vi "Main.vi"(11 "Module Admin":refnum<class "Delacor_lib_QMH_Module Admin.lvclass">) -> ()   [LabVIEW 2021, in "PS.lvlib"]
doc: "This template is based off of the Queued Message Handler design pattern and the Queued Message Handler project template that ships with LabVIEW.\n\nThe main difference is that the queue is private to this module and communication between modules is performed via Broadcast and Request events.\n\nRequest events are wrapped in public API methods and are handled in the Event Handling Loop (EHL) of this VI. Any module can register for Broadcast events sent by this module. The EHL generates messages based on user interface actions.\n\nThe Message Handling Loop (MHL) processes messages generated by the EHL, or by other messages. The messages are string values, so new messages can be added easily to the Message Cases case structure in the MHL. Each message cluster can also provide an optional value for Message Data, which is a variant that can be converted to whatever message-specific data is required.\n_____\nBased on Delacor QMH Project Template 5.0.0.82.\n\n<b>Note:</b> This VI was modified by the <b>Validate DQMH Module</b> tool to add a 'Panel Hidden' status updated broadcast to the Panel Close? event when External Launch = TRUE.\n\n<b>Note:</b> This VI was modified by the <b>Validate DQMH Module</b> tool to add a call to the Error Reported VI at the end of the 'Exit' MHL frame."
uses:
  PS.lvlib
  <vilib>/Delacor/Delacor QMH/Libraries/Module Admin_class/Delacor_lib_QMH_Module Admin.lvclass
  td_en_pstype.ctl
  Classes/PS/PS.lvclass
  <vilib>/Delacor/Delacor QMH/Libraries/Message Queue_class/Delacor_lib_QMH_Message Queue.lvclass/Delacor_lib_QMH_Message Queue.ctl
  Stop Argument--cluster.ctl
  <vilib>/Delacor/Delacor QMH/Libraries/Module Admin_class/Delacor_lib_QMH_Module Admin.lvclass/Delacor_lib_QMH_Module Admin.ctl
  Set Power Supply Argument--cluster.ctl
  Set Voltage Argument--cluster.ctl
  Set Current Argument--cluster.ctl
  Set Output Argument--cluster.ctl
  Open Argument--cluster.ctl
  Open (Reply Payload)--cluster.ctl
  Close Argument--cluster.ctl
  Close (Reply Payload)--cluster.ctl
  Get PS Data Argument--cluster.ctl
  Get PS Data (Reply Payload)--cluster.ctl
  Load in SubPane Argument--cluster.ctl
  UnLoad SubPane Argument--cluster.ctl
  <vilib>/Utility/miscctls.llb/LVPointTypeDef.ctl
  <vilib>/Delacor/Delacor QMH/Libraries/Message Queue_class/Delacor_lib_QMH_Enqueue Message (Single).vi
  <vilib>/Delacor/Delacor QMH/Libraries/Module Admin_class/Delacor_lib_QMH_Get External Launch.vi
  <vilib>/Utility/error.llb/Error Cluster From Error Code.vi
  <vilib>/ErrorRing/Error Ring.xnode
  <vilib>/Delacor/Delacor QMH/Libraries/Message Queue_class/Delacor_lib_QMH_Message Queue.lvclass
  Model/Model.lvlib
  <vilib>/DQMH Consortium/Lumos API/Libraries/SDV API/SDV API.lvlib
panel:
  in  "PS Type":T1
  out "Subpanel Ref":refnum<vi>
  in  "Set PS type":bool
  in  "Type":T1
  out "PS type":string
  in  "Get PS Data":bool
  in  "Current":dbl=0.8
  in  "Voltage":dbl=5.0
  out "Output?":bool
  out "Curr Read":dbl
  out "Volt Read":dbl
  in  "Enable Output":bool
  in  "Set Current":bool
  in  "Set Voltage":bool
  out "ModuleName":string
  in  "ExitMod":bool
  in  "Simulate MHL Error":bool
  in  "Simulate EHL Error":bool
  out "error out":errorcluster
  out "Status":string
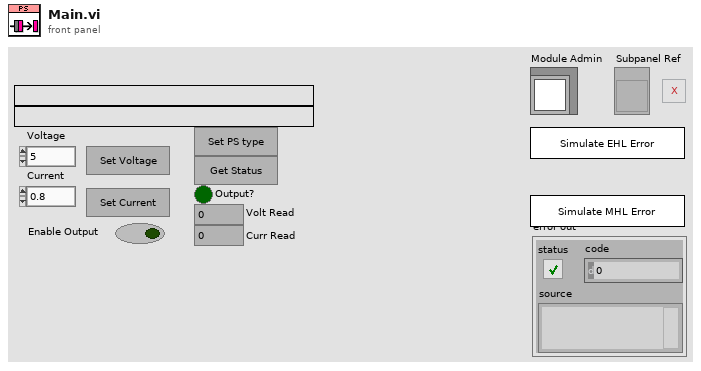
[diagram p1: front panel]
types:
  T1 = typedef "PS.lvlib/td_en_pstype.ctl" = enum16{"PS Simulated", "Keysight E3642A", "PS Test", "PS"}
  T2 = typedef "PS.lvlib/Request Events--cluster.ctl" = cluster{"Stop Module":refnum<user-event>, "Show Panel":refnum<user-event>, "Hide Panel":refnum<user-event>, "Get Module Execution Status":refnum<user-event>, "Show Diagram":refnum<user-event>, "Set Power Supply":refnum<user-event>, "Set Voltage":refnum<user-event>, "Set Current":refnum<user-event>, "Set Output":refnum<user-event>, "Open":refnum<user-event>, "Close":refnum<user-event>, "Get PS Data":refnum<user-event>, "Load in SubPane":refnum<user-event>, "UnLoad SubPane":refnum<user-event>}
  T3 = enum32{"invalid lock state", "Not Locked", "Locked (No Password)", "Password-protected"}
  T4 = typedef "PS.lvlib/Stop Argument--cluster.ctl" = cluster{"Origin":string, "Exit via Stop Module Req?":bool, "Wait for Module to stop?":bool}
  T5 = typedef "PS.lvlib/Set Power Supply Argument--cluster.ctl" = cluster{"Power Supply class":T1}
  T6 = typedef "PS.lvlib/Set Voltage Argument--cluster.ctl" = cluster{"Voltage":dbl}
  T7 = typedef "PS.lvlib/Set Current Argument--cluster.ctl" = cluster{"Curr":dbl}
  T8 = typedef "PS.lvlib/Set Output Argument--cluster.ctl" = cluster{"Output?":bool}
  T9 = typedef "PS.lvlib/Open Argument--cluster.ctl" = cluster{"Resource":string, "Wait Notifier":refnum<notifier>, "wait for reply":bool}
  T10 = typedef "PS.lvlib/Close Argument--cluster.ctl" = cluster{"Wait Notifier":refnum<notifier>, "wait for reply":bool}
  T11 = typedef "PS.lvlib/Get PS Data Argument--cluster.ctl" = cluster{"Wait Notifier":refnum<notifier>, "wait for reply":bool}
  T12 = typedef "PS.lvlib/Load in SubPane Argument--cluster.ctl" = cluster{"Subpanel Ref":refnum<vi>}
  T13 = typedef "PS.lvlib/UnLoad SubPane Argument--cluster.ctl" = cluster{"Subpanel Ref":refnum<vi>}
  T14 = typedef "LVPointTypeDef.ctl" = cluster{"Horizontal":i16, "Vertical":i16}
  T15 = enum32{"Invalid", "Standard", "Closed", "Hidden", "Minimized", "Maximized"}
  T16 = typedef "PS.lvlib/Open (Reply Payload)--cluster.ctl" = cluster{"error":errorcluster}
  T17 = typedef "PS.lvlib/Close (Reply Payload)--cluster.ctl" = cluster{"error":errorcluster}
  T18 = typedef "PS.lvlib/Get PS Data (Reply Payload)--cluster.ctl" = cluster{"Current":dbl, "Voltage":dbl, "Output?":bool, "error":errorcluster}
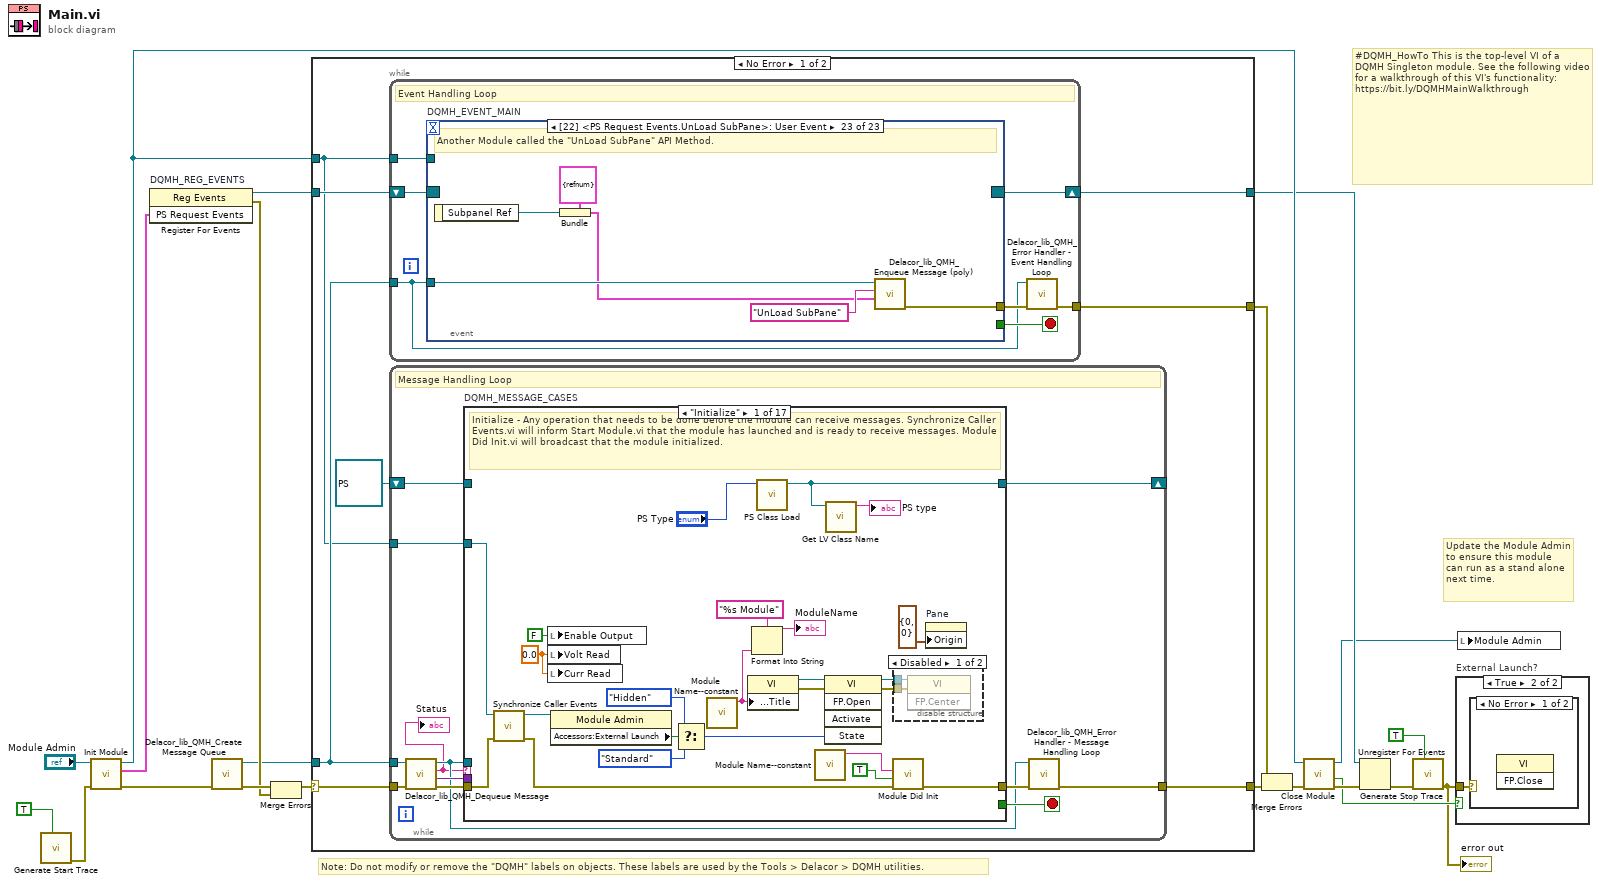
[diagram p0: block diagram]
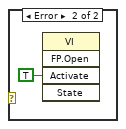
[diagram p3: hidden frame]
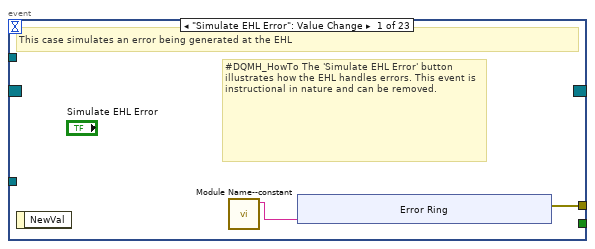
[diagram p4: hidden frame]
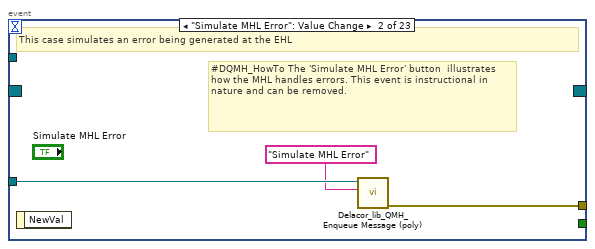
[diagram p5: hidden frame]
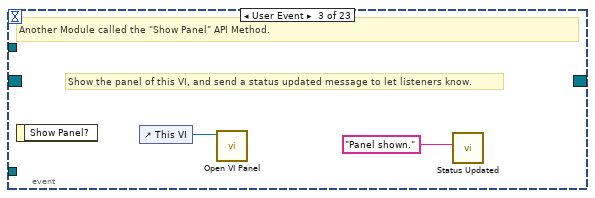
[diagram p6: hidden frame]
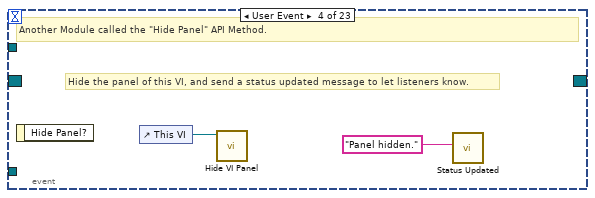
[diagram p7: hidden frame]
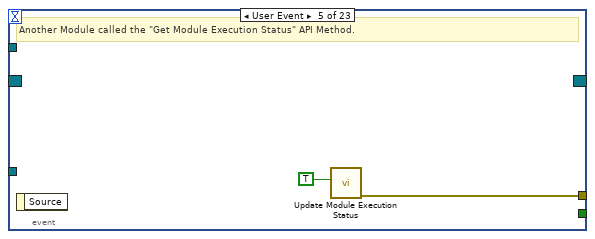
[diagram p8: hidden frame]
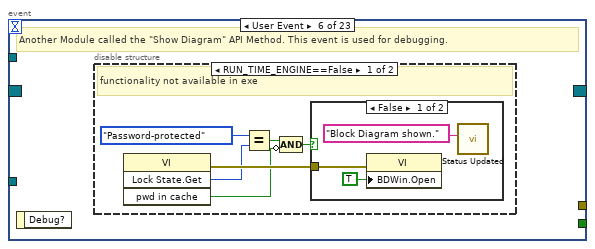
[diagram p9: hidden frame]
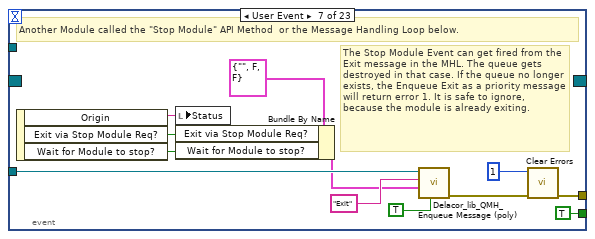
[diagram p12: hidden frame]
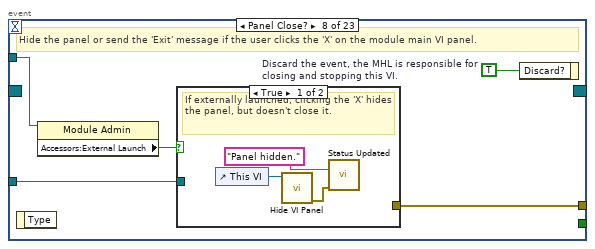
[diagram p13: hidden frame]
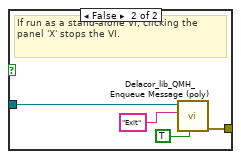
[diagram p14: hidden frame]
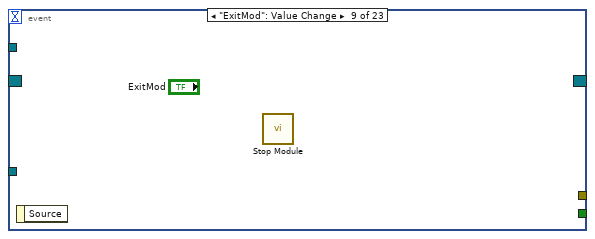
[diagram p15: hidden frame]
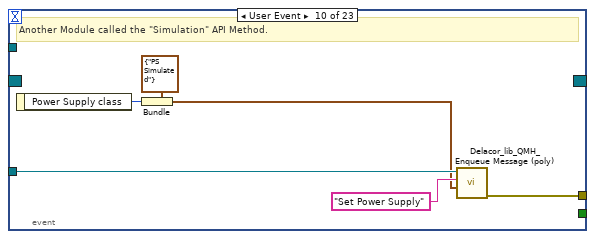
[diagram p16: hidden frame]
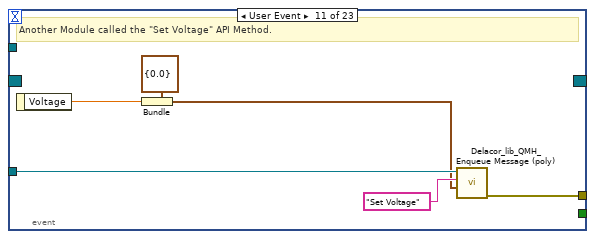
[diagram p17: hidden frame]
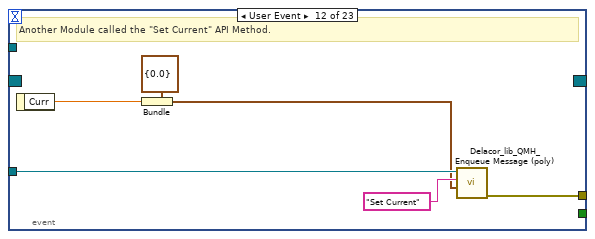
[diagram p18: hidden frame]
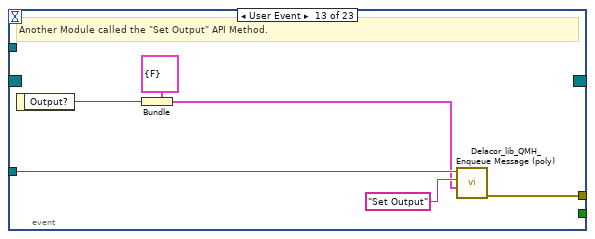
[diagram p19: hidden frame]
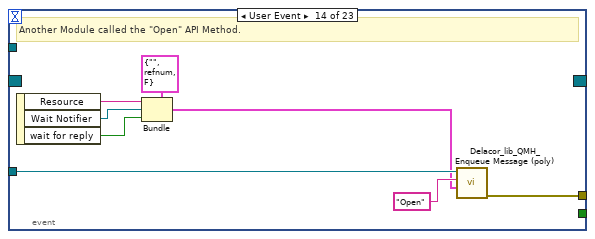
[diagram p20: hidden frame]
diagram:
  # "#DQMH_HowTo This is the top-level VI of a DQMH Singleton module. See the following video for a walkthrough of this VI's functionality: https://bit.ly/DQMHMainWalkthrough"
  # "Note: Do not modify or remove the \"DQMH\" labels on objects. These labels are used by the Tools > Delacor > DQMH utilities."
  # "Update the Module Admin to ensure this module can run as a stand alone next time."
  n1 = call <vilib>:"Generate Start Trace.vi"("Reply (F)"=TRUE) -> ("error out"=w4:errorcluster)  [unwired: 10 in]
  n2 = call "Init Module.vi"("error in (no error)"=w4, "Singleton Module Admin in"="Module Admin") -> ("error out"=w20:errorcluster, "PS Request Events"=w9:T2, "Singleton Module Admin out"=w12:refnum<class "Delacor_lib_QMH_Module Admin.lvclass">)  [unwired: 7 in]
  n3 = register-events "DQMH_REG_EVENTS"(w9) -> (reference out=w10:refnum<event-registration>, error out=w13:errorcluster)  [unwired: 2 in]
  n4 = call <vilib>:"Delacor_lib_QMH_Create Message Queue.vi"("error in"=w20) -> ("error out"=w15:errorcluster, "Message Queue"=w8:refnum<class "Delacor_lib_QMH_Message Queue.lvclass">)  [unwired: 9 in]
  n5 = Merge Errors(w15, w13) -> (w14:errorcluster)
  n6 = case shown="No Error" w14 {
    selector: w14 -> [w27 w374]
    tunnel: [w29 w373] -> w21
    tunnel: [w26 w379] -> w11
    tunnel: w10 -> [w25 w379]
    tunnel: w8 -> [w24 w372]
    tunnel: [w28 _] -> w18
    tunnel: w12 -> [w23 w375]
    frame No Error {
      n7 = while {
        tunnel: w24 -> [w30]
        shift-right: [w33] -> w26
        shift-left: w25 -> [w34]
        tunnel: [w35] -> w28
        tunnel: w23 -> [w31]
        stop <- w32 stop-if-true
        # "Event Handling Loop"
        n8 = event "DQMH_EVENT_MAIN" shown="[22] <PS Request Events.UnLoad SubPane>: User Event" {
          selector: w34 -> [_ _ _ _ _ _ _ _ _ _ _ _ _ _ _ _ _ _ _ _ _ _ _]
          dyn-events: [_ _ _ _ _ _ _ _ _ _ _ _ _ _ _ _ _ _ _ _ _ _ _] -> w33
          timeout: _ -> [_ _ _ _ _ _ _ _ _ _ _ _ _ _ _ _ _ _ _ _ _ _ _]
          tunnel: [_ _ _ _ _ _ TRUE ("Discard?") _ _ _ _ _ _ _ _ _ _ _ _ _ _ _ _] -> w32
          tunnel: w30 -> [_ w47 _ _ _ _ w71 w78 _ w93 w99 w105 w111 w119 w126 w133 _ _ _ _ _ w148 w154]
          tunnel: [w38 w48 _ _ w54 _ w74 w80 _ w89 w94 w100 w106 w112 w120 w127 w134 w137 w138 w140 _ w143 w149] -> w36
          tunnel: w31 -> [_ _ _ _ _ _ _ w77 _ _ _ _ _ _ _ _ _ _ _ _ _ _ _]
          event "Simulate EHL Error": Value Change {
            # "#DQMH_HowTo The 'Simulate EHL Error' button  illustrates how the EHL handles errors. This event is instructional in nature and can be removed."
            # "This case simulates an error being generated at the EHL"
            n9 = event-data() -> ()  [unwired: 1 in, 1 out]
            n10 = call "Module Name--constant.vi"() -> ("Module Name"=w37:string)  [unwired: 11 in]
            n11 = xnode ("Error Ring")("parameter 0"=w37) -> ("error out"=w38:errorcluster)
          }
          event "Simulate MHL Error": Value Change {
            # "#DQMH_HowTo The 'Simulate MHL Error' button  illustrates how the MHL handles errors. This event is instructional in nature and can be removed."
            # "This case simulates an error being generated at the EHL"
            n12 = event-data() -> ()  [unwired: 1 in, 1 out]
            n13 = call-poly <vilib>:"Delacor_lib_QMH_Enqueue Message (poly).vi"("Message"="Simulate MHL Error", "Message Queue in"=w47) -> ("error out"=w48:errorcluster)  [unwired: 8 in, 1 out]
          }
          event User Event {
            # "Show the panel of this VI, and send a status updated message to let listeners know."
            # "Another Module called the \"Show Panel\" API Method."
            n14 = event-data() -> ()  [unwired: 1 in, 1 out]
            n15 = control-ref of="This VI"() -> (w50:refnum<vi>)
            n16 = call "Open VI Panel.vi"("VI"=w50) -> ()  [unwired: 10 in, 1 out]
            n17 = call "Status Updated.vi"("Status"="Panel shown." ("format string")) -> ()  [unwired: 10 in, 1 out]
          }
          event User Event {
            # "Hide the panel of this VI, and send a status updated message to let listeners know."
            # "Another Module called the \"Hide Panel\" API Method."
            n18 = event-data() -> ()  [unwired: 1 in, 1 out]
            n19 = control-ref of="This VI"() -> (w52:refnum<vi>)
            n20 = call "Hide VI Panel.vi"("VI"=w52) -> ()  [unwired: 10 in, 1 out]
            n21 = call "Status Updated.vi"("Status"="Panel hidden." ("format string")) -> ()  [unwired: 10 in, 1 out]
          }
          event User Event {
            # "Another Module called the \"Get Module Execution Status\" API Method."
            n22 = event-data() -> ()  [unwired: 1 in, 1 out]
            n23 = call "Update Module Execution Status.vi"("Running?"=TRUE) -> ("error out"=w54:errorcluster)  [unwired: 10 in]
          }
          event User Event {
            # "Another Module called the \"Show Diagram\" API Method. This event is used for debugging."
            n24 = event-data() -> ()  [unwired: 1 in, 1 out]
            n25 = disable-structure "Conditional Disable Structure" shown="RUN_TIME_ENGINE==False" {
              frame condition #0 (active) {
                # "functionality not available in exe"
                n26 = invoke on="Invoke Node" class="VI" method="Lock State.Get"() -> (error out=w60:errorcluster, "Get Lock State"=w59:T3, "pwd in cache"=w56:bool)  [unwired: 4 in, 1 out]
                n27 = Equal?(x=T3."Password-protected", y=w59) -> (x = y?=w57:bool)
                n28 = Compound Arithmetic op=AND(w57, invert w56) -> (w55:bool)
                n29 = case shown="False" w55 {
                  tunnel: w60 -> [w63 _]
                  frame False {
                    n30 = property on="Property Node" class="VI"(error in=w63, "BDWin.Open"=TRUE ("Block Diagram Window:Open")) -> ()  [unwired: 1 in, 2 out]
                    n31 = call "Status Updated.vi"("Status"="Block Diagram shown." ("format string")) -> ()  [unwired: 10 in, 1 out]
                  }
                  frame True {
                    # "Password-protected VI, and the password is not in the cache. Do not show the diagram."
                  }
                }
              }
              frame condition #1 {
              }
            }
          }
          event User Event {
            # "The Stop Module Event can get fired from the Exit message in the MHL. The queue gets destroyed in that case. If the queue no longer exists, the Enqueue Exit as a priority message will return error 1. It is safe to ignore, because the module is already exiting."
            # "Another Module called the \"Stop Module\" API Method  or the Message Handling Loop below."
            n32 = event-data() -> ("Origin"=w70:string, "Exit via Stop Module Req?"=w66:bool, "Wait for Module to stop?"=w65:bool)  [unwired: 1 in]
            n33 = local write "Status"(w70) -> ()
            n34 = Bundle By Name(cluster=T4 {"Origin"="", "Exit via Stop Module Req?"=FALSE, "Wait for Module to stop?"=FALSE} ("Stop Argument"), "Exit via Stop Module Req?"=w66, "Wait for Module to stop?"=w65) -> (w64:T4)
            n35 = call-poly <vilib>:"Delacor_lib_QMH_Enqueue Message (poly).vi"("Priority Message? (F)"=TRUE, "Message Data"=w64, "Message"="Exit", "Message Queue in"=w71) -> ("error out"=w75:errorcluster)  [unwired: 6 in, 1 out]
            n36 = call <vilib>:"Clear Errors.vi"("error in (no error)"=w75, "specific error code to clear (0: all)"=1) -> ("error out"=w74:errorcluster)  [unwired: 4 in, 1 out]
          }
          event Panel Close? {
            w79 = TRUE  # Discard the event, the MHL is responsible for closing and stopping this VI.
            # "Hide the panel or send the 'Exit' message if the user clicks the 'X' on the module main VI panel."
            n37 = event-data() -> ()  [unwired: 1 in, 1 out]
            n38 = property on="Property Node" class="Module Admin"(reference=w77) -> ("Accessors:External Launch"=w76:bool)  [unwired: 1 in, 2 out]
            n39 = case shown="True" w76 {
              tunnel: w78 -> [_ w86]
              tunnel: [_ w87] -> w80
              frame True {
                # "If externally launched, clicking the 'X' hides the panel, but doesn't close it."
                n40 = control-ref of="This VI"() -> (w83:refnum<vi>)
                n41 = call "Hide VI Panel.vi"("VI"=w83) -> ("error out"=w81:errorcluster)  [unwired: 10 in]
                n42 = call "Status Updated.vi"("error in (no error)"=w81, "Status"="Panel hidden.") -> ()  [unwired: 9 in, 1 out]
              }
              frame False {
                # "If run as a stand-alone VI, clicking the panel 'X' stops the VI."
                n43 = call-poly <vilib>:"Delacor_lib_QMH_Enqueue Message (poly).vi"("Priority Message? (F)"=TRUE, "Message"="Exit", "Message Queue in"=w86) -> ("error out"=w87:errorcluster)  [unwired: 7 in, 1 out]
              }
            }
            n44 = event-data ("Event Filter Node")("Discard?"=w79) -> ()  [unwired: 1 in, 1 out]
          }
          event "ExitMod": Value Change {
            n45 = event-data() -> ()  [unwired: 1 in, 1 out]
            n46 = call "Stop Module.vi"() -> ()  [unwired: 11 in, 1 out]
          }
          event User Event {
            # "Another Module called the \"Simulation\" API Method."
            n47 = event-data() -> ("Power Supply class"=w88:T1)  [unwired: 1 in]
            n48 = Bundle(cluster=T5 {"Power Supply class"=enum."PS Simulated"} ("Simulation Argument"), "Power Supply class"=w88) -> (w90:T5)
            n49 = call-poly <vilib>:"Delacor_lib_QMH_Enqueue Message (poly).vi"("Message Data"=w90, "Message"="Set Power Supply", "Message Queue in"=w93) -> ("error out"=w89:errorcluster)  [unwired: 7 in, 1 out]
          }
          event User Event {
            # "Another Module called the \"Set Voltage\" API Method."
            n50 = event-data() -> ("Voltage"=w95:dbl)  [unwired: 1 in]
            n51 = Bundle(cluster=T6 {"Voltage"=0.0} ("Set Voltage Argument"), "Voltage"=w95) -> (w96:T6)
            n52 = call-poly <vilib>:"Delacor_lib_QMH_Enqueue Message (poly).vi"("Message Data"=w96, "Message"="Set Voltage", "Message Queue in"=w99) -> ("error out"=w94:errorcluster)  [unwired: 7 in, 1 out]
          }
          event User Event {
            # "Another Module called the \"Set Current\" API Method."
            n53 = event-data() -> ("Curr"=w101:dbl)  [unwired: 1 in]
            n54 = Bundle(cluster=T7 {"Curr"=0.0} ("Set Current Argument"), "Curr"=w101) -> (w102:T7)
            n55 = call-poly <vilib>:"Delacor_lib_QMH_Enqueue Message (poly).vi"("Message Data"=w102, "Message"="Set Current", "Message Queue in"=w105) -> ("error out"=w100:errorcluster)  [unwired: 7 in, 1 out]
          }
          event User Event {
            # "Another Module called the \"Set Output\" API Method."
            n56 = event-data() -> ("Output?"=w107:bool)  [unwired: 1 in]
            n57 = Bundle(cluster=T8 {"Output?"=FALSE} ("Set Output Argument"), "Output?"=w107) -> (w108:T8)
            n58 = call-poly <vilib>:"Delacor_lib_QMH_Enqueue Message (poly).vi"("Message Data"=w108, "Message"="Set Output", "Message Queue in"=w111) -> ("error out"=w106:errorcluster)  [unwired: 7 in, 1 out]
          }
          event User Event {
            # "Another Module called the \"Open\" API Method."
            n59 = event-data() -> ("Resource"=w115:string, "Wait Notifier"=w114:refnum<notifier>, "wait for reply"=w113:bool)  [unwired: 1 in]
            n60 = Bundle(cluster=T9 {"Resource"="", "Wait Notifier"=refnum, "wait for reply"=FALSE} ("Open Argument"), "Resource"=w115, "Wait Notifier"=w114, "wait for reply"=w113) -> (w116:T9)
            n61 = call-poly <vilib>:"Delacor_lib_QMH_Enqueue Message (poly).vi"("Message Data"=w116, "Message"="Open", "Message Queue in"=w119) -> ("error out"=w112:errorcluster)  [unwired: 7 in, 1 out]
          }
          event User Event {
            # "Another Module called the \"Close\" API Method."
            n62 = event-data() -> ("Wait Notifier"=w122:refnum<notifier>, "wait for reply"=w121:bool)  [unwired: 1 in]
            n63 = Bundle(cluster=T10 {"Wait Notifier"=refnum, "wait for reply"=FALSE} ("Close Argument"), "Wait Notifier"=w122, "wait for reply"=w121) -> (w123:T10)
            n64 = call-poly <vilib>:"Delacor_lib_QMH_Enqueue Message (poly).vi"("Message Data"=w123, "Message"="Close", "Message Queue in"=w126) -> ("error out"=w120:errorcluster)  [unwired: 7 in, 1 out]
          }
          event User Event {
            # "Another Module called the \"Get Module Data\" API Method."
            n65 = event-data() -> ("Wait Notifier"=w129:refnum<notifier>, "wait for reply"=w128:bool)  [unwired: 1 in]
            n66 = Bundle(cluster=T11 {"Wait Notifier"=refnum, "wait for reply"=FALSE} ("Get Module Data Argument"), "Wait Notifier"=w129, "wait for reply"=w128) -> (w130:T11)
            n67 = call-poly <vilib>:"Delacor_lib_QMH_Enqueue Message (poly).vi"("Message Data"=w130, "Message"="Get PS Data", "Message Queue in"=w133) -> ("error out"=w127:errorcluster)  [unwired: 7 in, 1 out]
          }
          event "Enable Output": Value Change {
            n68 = event-data() -> ()  [unwired: 1 in, 1 out]
            n69 = call "Set Output.vi"("Output?"="Enable Output") -> ("error out"=w134:errorcluster)  [unwired: 10 in]
          }
          event "Set PS type": Value Change {
            n70 = event-data() -> ()  [unwired: 1 in, 1 out]
            n71 = call "Set Power Supply.vi"("Power Supply class"="Type") -> ("error out"=w137:errorcluster)  [unwired: 10 in]
          }
          event "Set Voltage": Value Change {
            n72 = event-data() -> ()  [unwired: 1 in, 1 out]
            n73 = call "Set Voltage.vi"("Voltage"="Voltage") -> ("error out"=w138:errorcluster)  [unwired: 10 in]
          }
          event "Set Current": Value Change {
            n74 = event-data() -> ()  [unwired: 1 in, 1 out]
            n75 = call "Set Current.vi"("Curr"="Current") -> ("error out"=w140:errorcluster)  [unwired: 10 in]
          }
          event "Get PS Data": Value Change {
            # "Another Module called the \"Get Module Data\" API Method."
            n76 = event-data() -> ()  [unwired: 1 in, 2 out]
            n77 = call "Get PS Data.vi"("wait for reply (T)"=FALSE) -> ()  [unwired: 8 in, 3 out]
          }
          event User Event {
            # "Another Module called the \"Load in SubPane\" API Method."
            n78 = event-data() -> ("Subpanel Ref"=w144:refnum<vi>)  [unwired: 1 in]
            n79 = Bundle(cluster=T12 {"Subpanel Ref"=refnum} ("Load in SubPane Argument"), "Subpanel Ref"=w144) -> (w145:T12)
            n80 = call-poly <vilib>:"Delacor_lib_QMH_Enqueue Message (poly).vi"("Message Data"=w145, "Message"="Load in SubPane", "Message Queue in"=w148) -> ("error out"=w143:errorcluster)  [unwired: 7 in, 1 out]
          }
          event User Event {
            # "Another Module called the \"UnLoad SubPane\" API Method."
            n81 = event-data() -> ("Subpanel Ref"=w150:refnum<vi>)  [unwired: 1 in]
            n82 = Bundle(cluster=T13 {"Subpanel Ref"=refnum} ("UnLoad SubPane Argument"), "Subpanel Ref"=w150) -> (w151:T13)
            n83 = call-poly <vilib>:"Delacor_lib_QMH_Enqueue Message (poly).vi"("Message Data"=w151, "Message"="UnLoad SubPane", "Message Queue in"=w154) -> ("error out"=w149:errorcluster)  [unwired: 7 in, 1 out]
          }
        }
        n84 = call-dynamic "Delacor_lib_QMH_Error Handler - Event Handling Loop.vi"("error in"=w36, "Message Queue in"=w30) -> ("dup error in"=w35:errorcluster)  [unwired: 8 in, 1 out]
      }
      n85 = while {
        tunnel: w24 -> [w160]
        shift-right: [w155] -> _
        shift-left: refnum<class "PS.lvclass"> refnum ("PS.lvclass") -> [w157]
        tunnel: w27 -> [w165]
        tunnel: [w163] -> w29
        tunnel: w23 -> [w158]
        stop <- w162 stop-if-true
        # "Message Handling Loop"
        n86 = call-dynamic "Delacor_lib_QMH_Dequeue Message.vi"("error in"=w165, "Message Queue in"=w160) -> ("error out"=w164:errorcluster, "Message Data"=w161:variant, "Message"=w156:string, "Message Queue out"=w159:refnum<class "Delacor_lib_QMH_Message Queue.lvclass">)  [unwired: 6 in]
        "Status" <- w156
        n87 = case "DQMH_MESSAGE_CASES" shown="\"Initialize\"" w156 {
          selector: w156 -> [_ _ _ w215 w226 w239 w254 _ _ _ _ _ _ _ _ _ w359]
          tunnel: w159 -> [_ _ _ _ _ _ _ _ _ _ _ _ _ _ w327 w352 _]
          tunnel: w164 -> [w189 w194 w207 w220 w232 w244 w259 w272 w290 w300 w307 w310 w312 w317 w334 w357 w361]
          tunnel: [w187 w194 w199 w219 w231 w243 w258 w263 w281 w298 w305 w309 w312 w316 w330 w354 w362] -> w166
          tunnel: w157 -> [_ w193 w196 _ w227 w237 w247 w261 w279 w299 w306 w308 w311 w314 w329 w351 w360]
          tunnel: [w168 w193 w197 w211 w224 w236 w248 w260 w278 w299 w306 w308 w311 w314 w329 w351 w360] -> w155
          tunnel: [_ _ _ _ _ _ _ _ _ _ _ _ _ _ _ w350 _] -> w162
          tunnel: w161 -> [_ _ w205 w218 w230 w242 w257 w270 w288 w297 w304 _ _ _ w328 w349 _]
          tunnel: w158 -> [w181 _ _ _ _ _ _ _ _ _ _ _ _ _ w326 w344 _]
          frame "Initialize" {
            w171 = 0.0 ("Volt Read")
            # "Initialize - Any operation that needs to be done before the module can receive messages. Synchronize Caller Events.vi will inform Start Module.vi that the module has launched and is ready to receive messages. Module Did Init.vi will broadcast that the module initialized."
            n88 = call "Synchronize Caller Events.vi"("error in (no error)"=w189, "Singleton Module Admin in"=w181) -> ("error out"=w188:errorcluster, "Singleton Module Admin out"=w178:refnum<class "Delacor_lib_QMH_Module Admin.lvclass">)  [unwired: 8 in]
            n89 = local write "Enable Output"(FALSE ("Enable Output")) -> ()
            n90 = local write "Volt Read"(w171) -> ()
            n91 = local write "Curr Read"(w171) -> ()
            n92 = property on="Property Node" class="Module Admin"(reference=w178) -> ("Accessors:External Launch"=w185:bool)  [unwired: 1 in, 2 out]
            n93 = Select(t=T15."Hidden" ("State"), s=w185, f=T15."Standard" ("State")) -> (s? t:f=w182:T15)
            n94 = call "Module Name--constant.vi"() -> ("Module Name"=w176:string)  [unwired: 11 in]
            n95 = property on="Property Node" class="VI"("Front Panel.Title"=w176) -> (reference out=w173:refnum<vi>, error out=w190:errorcluster)  [unwired: 2 in]
            n96 = Format Into String(format string="%s Module", w176) -> (resulting string=→"ModuleName":string)  [unwired: 2 in, 1 out]
            n97 = call "PS Class Load.vi"("PS Type"="PS Type") -> ("PS.lvclass"=w168:refnum<class "PS.lvclass">)  [unwired: 9 in, 1 out]
            n98 = call "Module Name--constant.vi"() -> ("Module Name"=w179:string)  [unwired: 11 in]
            n99 = invoke on="Invoke Node" class="VI" method="FP.Open"(reference=w173, error in=w190, "State"=w182) -> (reference out=w186:refnum<vi>, error out=w167:errorcluster)  [unwired: 2 in, 3 out]
            n100 = call <vilib>:"Get LV Class Name.vi"("object"=w168) -> ("class name"=→"PS type":string)  [unwired: 9 in, 1 out]
            n101 = call "Module Did Init.vi"("error in (no error)"=w188, "Initialized?"=TRUE, "Origin"=w179) -> ("error out"=w187:errorcluster)  [unwired: 8 in]
            n102 = disable-structure "Diagram Disable Structure" shown="Disabled" {
              disable-tunnel: w167 -> [w192 _]
              disable-tunnel: w186 -> [w191 _]
              frame Disabled {
                n103 = invoke on="Invoke Node" class="VI" method="FP.Center"(reference=w191, error in=w192) -> ()  [unwired: 1 in, 3 out]
              }
              frame Enabled {
              }
            }
            n104 = property on="Pane" class="Pane"("Origin"=T14 {"Horizontal"=0, "Vertical"=0}) -> ()  [unwired: 2 in, 2 out]
          }
          frame "--- Module Specific ---" {
            # "Separator -- The following cases handle messages specific to this Module."
          }
          frame "Open" {
            # "#FIx Add Resource"
            n105 = Variant To Data(error in=w207, type=T9 {"Resource"="", "Wait Notifier"=refnum, "wait for reply"=FALSE} ("Open Argument"), Variant=w205) -> (data=w195:T9, error out=w206:errorcluster)
            n106 = Unbundle By Name(w195) -> ()  [unwired: 1 out]
            n107 = call-dynamic "Open.vi"("PS in"=w196) -> ("error out"=w198:errorcluster, "PS out"=w197:refnum<class "PS.lvclass">)  [unwired: 9 in]
            n108 = Unbundle By Name(w195) -> ("Wait Notifier"=w203:refnum<notifier>, "wait for reply"=w202:bool)
            n109 = Merge Errors(w206, w198) -> (w199:errorcluster)
            n110 = Bundle By Name(cluster=T16 {"error"={"status"=FALSE, "code"=0, "source"=""}} ("Open (Reply Payload)"), "error"=w198) -> (w201:T16)
            n111 = case shown="True" w202 {
              tunnel: w203 -> [_ w209]
              tunnel: w201 -> [_ w208]
              frame False {
              }
              frame True {
                n112 = Send Notification(notification=w208, notifier=w209) -> ()  [unwired: 1 in, 2 out]
              }
            }
          }
          frame "Set Power Supply" {
            # "#Fix Looses data when switching"
            # "This will change Module into Simulation Mode"
            n113 = Variant To Data(error in=w220, type=T5 {"Power Supply class"=enum."PS Simulated"} ("Simulation Argument"), Variant=w218) -> (data=w216:T5, error out=w219:errorcluster)
            n114 = Unbundle By Name(w216) -> ("Power Supply class"=w213:T1)
            n115 = call "PS Class Load.vi"("PS Type"=w213) -> ("PS.lvclass"=w212:refnum<class "PS.lvclass">)  [unwired: 9 in, 1 out]
            n116 = Format Into String(format string="%s: %s", w215, w213) -> (resulting string=w210:string)  [unwired: 2 in, 1 out]
            n117 = call-dynamic "Set Status.vi"("Status"=w210, "PS in"=w212) -> ("PS out"=w211:refnum<class "PS.lvclass">)  [unwired: 8 in, 1 out]
          }
          frame "Set Voltage" {
            n118 = Variant To Data(error in=w232, type=T6 {"Voltage"=0.0} ("Set Voltage Argument"), Variant=w230) -> (data=w228:T6, error out=w231:errorcluster)
            n119 = Unbundle By Name(w228) -> ("Voltage"=w223:dbl)
            n120 = Format Into String(format string="%s: %f", w226, w223) -> (resulting string=w221:string)  [unwired: 2 in, 1 out]
            n121 = call-dynamic "Set Status.vi"("Status"=w221, "PS in"=w227) -> ("PS out"=w222:refnum<class "PS.lvclass">)  [unwired: 8 in, 1 out]
            n122 = call-dynamic "Set Voltage.vi"("Voltage"=w223, "PS in"=w222) -> ("PS out"=w224:refnum<class "PS.lvclass">)  [unwired: 8 in, 1 out]
          }
          frame "Set Current" {
            # "Sets PS Current Limit"
            n123 = Variant To Data(error in=w244, type=T7 {"Curr"=0.0} ("Set Current Argument"), Variant=w242) -> (data=w240:T7, error out=w243:errorcluster)
            n124 = Unbundle By Name(w240) -> ("Curr"=w234:dbl)
            n125 = Format Into String(format string="%s: %f", w239, w234) -> (resulting string=w233:string)  [unwired: 2 in, 1 out]
            n126 = call-dynamic "Set Status.vi"("Status"=w233, "PS in"=w237) -> ("PS out"=w235:refnum<class "PS.lvclass">)  [unwired: 8 in, 1 out]
            n127 = call-dynamic "Set Current.vi"("Current"=w234, "PS in"=w235) -> ("PS out"=w236:refnum<class "PS.lvclass">)  [unwired: 8 in, 1 out]
          }
          frame "Set Output" {
            # "Enables or Disables PS output"
            n128 = Variant To Data(error in=w259, type=T8 {"Output?"=FALSE} ("Set Output Argument"), Variant=w257) -> (data=w255:T8, error out=w258:errorcluster)
            n129 = Unbundle By Name(w255) -> ("Output?"=w252:bool)
            n130 = Select(t="True", s=w252, f="False") -> (s? t:f=w251:string)
            n131 = Format Into String(format string="%s: %s", w254, w251) -> (resulting string=w245:string)  [unwired: 2 in, 1 out]
            n132 = call-dynamic "Set Status.vi"("Status"=w245, "PS in"=w247) -> ("PS out"=w246:refnum<class "PS.lvclass">)  [unwired: 8 in, 1 out]
            n133 = call-dynamic "Set Output.vi"("Enable?"=w252, "PS in"=w246) -> ("PS out"=w248:refnum<class "PS.lvclass">)  [unwired: 8 in, 1 out]
          }
          frame "Close" {
            n134 = Variant To Data(error in=w272, type=T10 {"Wait Notifier"=refnum, "wait for reply"=FALSE} ("Close Argument"), Variant=w270) -> (data=w268:T10, error out=w271:errorcluster)
            n135 = call-dynamic "Close.vi"("PS in"=w261) -> ("error out"=w262:errorcluster, "PS out"=w260:refnum<class "PS.lvclass">)  [unwired: 9 in]
            n136 = Unbundle By Name(w268) -> ("Wait Notifier"=w267:refnum<notifier>, "wait for reply"=w266:bool)
            n137 = Bundle By Name(cluster=T17 {"error"={"status"=FALSE, "code"=0, "source"=""}} ("Close (Reply Payload)"), "error"=w262) -> (w265:T17)
            n138 = case shown="True" w266 {
              tunnel: w267 -> [_ w274]
              tunnel: w265 -> [_ w273]
              frame False {
              }
              frame True {
                n139 = Send Notification(notification=w273, notifier=w274) -> ()  [unwired: 1 in, 2 out]
              }
            }
            n140 = Merge Errors(w271, w262) -> (w263:errorcluster)
          }
          frame "Get PS Data" {
            n141 = Variant To Data(error in=w290, type=T11 {"Wait Notifier"=refnum, "wait for reply"=FALSE} ("Get Module Data Argument"), Variant=w288) -> (data=w286:T11, error out=w289:errorcluster)
            n142 = call-dynamic "Get Curr and Volt.vi"("PS in"=w279) -> ("PS out"=w278:refnum<class "PS.lvclass">, "Voltage"=w277:dbl, "Current"=w276:dbl, "Output?"=w275:bool, "error out"=w280:errorcluster)  [unwired: 10 in]
            "Volt Read" <- w277
            "Curr Read" <- w276
            "Output?" <- w275
            n143 = Unbundle By Name(w286) -> ("Wait Notifier"=w285:refnum<notifier>, "wait for reply"=w284:bool)
            n144 = Bundle By Name(cluster=T18 {"Current"=0.0, "Voltage"=0.0, "Output?"=FALSE, "error"={"status"=FALSE, "code"=0, "source"=""}} ("Get Module Data (Reply Payload)"), "Voltage"=w277, "Current"=w276, "Output?"=w275, "error"=w280) -> (w283:T18)
            n145 = Merge Errors(w289, w280) -> (w281:errorcluster)
            n146 = case shown="True" w284 {
              tunnel: w285 -> [_ w292]
              tunnel: w283 -> [_ w291]
              frame False {
              }
              frame True {
                n147 = Send Notification(notification=w291, notifier=w292) -> ()  [unwired: 1 in, 2 out]
              }
            }
          }
          frame "Load in SubPane" {
            n148 = Variant To Data(error in=w300, type=T12 {"Subpanel Ref"=refnum} ("Load in SubPane Argument"), Variant=w297) -> (data=w295:T12, error out=w298:errorcluster)
            n149 = Unbundle By Name(w295) -> ("Subpanel Ref"=w293:refnum<vi>)
            "Subpanel Ref" <- w293
            n150 = control-ref of="This VI"() -> (w294:refnum<vi>)
            n151 = call "Insert SubPanl.vi"("VI Ref"=w294, "Subpanel Ref"=w293) -> ()  [unwired: 9 in, 1 out]
          }
          frame "UnLoad SubPane" {
            n152 = Variant To Data(error in=w307, type=T13 {"Subpanel Ref"=refnum} ("UnLoad SubPane Argument"), Variant=w304) -> (data=w302:T13, error out=w305:errorcluster)
            n153 = Unbundle By Name(w302) -> ("Subpanel Ref"=w301:refnum<vi>)
            n154 = call "Remove SubPanel.vi"("Subpanel Ref"=w301) -> ()  [unwired: 10 in, 1 out]
          }
          frame "---Copy This Frame---" {
            # "Duplicate this frame when creating new messages.  Change this comment in the duplicated frame to describe this message."
            n155 = Merge Errors(w310) -> (w309:errorcluster)
          }
          frame "--- Exit and Error Handling---" {
            # "Separator - The following cases handle errors and exit messages."
          }
          frame "Simulate MHL Error" {
            # "#DQMH_HowTo The 'Simulate MHL Error' button  illustrates how the MHL handles errors. This event is instructional in nature and can be removed."
            # "Simulate an error occurring at the MHL"
            n156 = call "Module Name--constant.vi"() -> ("Module Name"=w313:string)  [unwired: 11 in]
            n157 = xnode ("Error Ring")("parameter 0"=w313) -> ("error out"=w315:errorcluster)
            n158 = Merge Errors(w317, w315) -> (w316:errorcluster)
          }
          frame "Error" {
            # "#CodeRecommended - If you ever change the name of this \"Error\" message, you'll need to update the name in the Check Loop Error.vi as well."
            # "#CodeRecommended - If the module is running in standalone mode (External Launch = FALSE), this code will pop up an error dialog and call the 'Exit' message if an error occurs. Add more fine-grained error handling here."
            # "Error - Check the error message data and respond accordingly. This message is sent by the \"Error Handler\" VIs at the end of each loop in this application."
            n159 = property on="Property Node" class="Module Admin"(reference=w326) -> ("Accessors:External Launch"=w325:bool)  [unwired: 1 in, 2 out]
            n160 = Variant To Data(error in=w334, type=errorcluster {"status"=FALSE, "code"=0, "source"=""} ("error constant"), Variant=w328) -> (data=w335:errorcluster, error out=w332:errorcluster)
            n161 = call "Error Reported.vi"("Error"=w335) -> ()  [unwired: 10 in, 1 out]
            n162 = case shown="False" w325 {
              tunnel: [w340 _] -> w331
              tunnel: w327 -> [w338 _]
              tunnel: w335 -> [w339 _]
              frame False {
                # "If the module is running standalone, then pop up an error dialog and call the \"Exit\" message."
                n163 = call <vilib>:"Simple Error Handler.vi"("error in (no error)"=w339) -> ()  [unwired: 4 in, 5 out]
                n164 = call-poly <vilib>:"Delacor_lib_QMH_Enqueue Message (poly).vi"("Priority Message? (F)"=TRUE, "Message"="Exit", "Message Queue in"=w338) -> ("error out"=w340:errorcluster)  [unwired: 7 in, 1 out]
              }
              frame True {
                # "If the module was launched externally, calling the Error Reported broadcast VI is the only action performed by the \"Error\" message. The module's caller can then process the error appropriately."
              }
            }
            n165 = Merge Errors(w332, w331) -> (w330:errorcluster)
            n166 = local write "error out"(w330) -> ()
          }
          frame "Exit" {
            w348 = 91  # 91: not all Exit messages will have an argument
            w350 = TRUE  # Stop the VI
            # "Release the message queue reference"
            # "Exit - Exit the application."
            n167 = Variant To Data(error in=w357, type=T4 {"Origin"="", "Exit via Stop Module Req?"=FALSE, "Wait for Module to stop?"=FALSE} ("Stop Argument"), Variant=w349) -> (data=w346:T4, error out=w353:errorcluster)
            n168 = call <vilib>:"Clear Errors.vi"("error in (no error)"=w353, "specific error code to clear (0: all)"=w348) -> ("error out"=w356:errorcluster)  [unwired: 4 in, 1 out]
            n169 = local read "Subpanel Ref"() -> (w342:refnum<vi>)
            n170 = control-ref of="This VI"() -> (w345:refnum<vi>)
            n171 = call "Remove SubPanel.vi"("Subpanel Ref"=w342) -> ("error out"=w341:errorcluster)  [unwired: 10 in]
            n172 = call-dynamic "Delacor_lib_QMH_Release Message Queue.vi"("error in"=w356, "Message Queue"=w352) -> ("error out"=w355:errorcluster)  [unwired: 9 in]
            n173 = call "Handle Exit.vi"("error in (no error)"=w341, "Stop Argument"=w346, "Admin in"=w344, "VI reference"=w345) -> ("error out"=w343:errorcluster)  [unwired: 6 in, 1 out]
            n174 = Merge Errors(w355, w343) -> (w354:errorcluster)
            n175 = call "Error Reported.vi"("Error"=w354) -> ()  [unwired: 10 in, 1 out]
          }
          frame Default {
            # "'Default' case only runs if there is a message that isn't defined in any of the other cases.  Output a programming error."
            n176 = call "Module Name--constant.vi"() -> ("Module Name"=w358:string)  [unwired: 11 in]
            n177 = xnode ("Error Ring")("parameter 0"=w359, "parameter 1"=w358) -> ("error out"=w363:errorcluster)
            n178 = Merge Errors(w361, w363) -> (w362:errorcluster)
          }
        }
        n179 = call-dynamic "Delacor_lib_QMH_Error Handler - Message Handling Loop.vi"("error in"=w166, "Message Queue in"=w159) -> ("dup error in"=w163:errorcluster)  [unwired: 8 in, 1 out]
      }
    }
    frame Error {
      # "Synchronize Caller Events.vi will inform Start Module.vi that the module has launched and will let the code calling Start Module.vi register for broadcasts and would permit the caller receive the broadcast that an error occurred at launch time."
      n180 = call-dynamic "Delacor_lib_QMH_Release Message Queue.vi"("error in"=w374, "Message Queue"=w372) -> ("error out"=w373:errorcluster)  [unwired: 9 in]
      n181 = call "Synchronize Caller Events.vi"("Singleton Module Admin in"=w375) -> ("error out"=w380:errorcluster)  [unwired: 9 in, 1 out]
      n182 = call "Module Name--constant.vi"() -> ("Module Name"=w378:string)  [unwired: 11 in]
      n183 = Format Into String(format string="An error occurred during initialization. %s is no longer running.", w378) -> (resulting string=w376:string)  [unwired: 2 in, 1 out]
      n184 = Merge Errors(w373, w380) -> (w381:errorcluster)
      n185 = call "Error Reported.vi"("Additional Information"=w376, "Error"=w381) -> ()  [unwired: 9 in, 1 out]
    }
  }
  n186 = Merge Errors(w18, w21) -> (w17:errorcluster)
  n187 = call "Close Module.vi"("error in (no error)"=w17, "Module Admin in"=w12) -> ("error out"=w19:errorcluster, "External Launch"=w5:bool, "Module Admin out"=w6:refnum<class "Delacor_lib_QMH_Module Admin.lvclass">)  [unwired: 7 in]
  n188 = Unregister For Events(event registration refnum=w11, error in=w19) -> (error out=w16:errorcluster)
  n189 = call <vilib>:"Generate Stop Trace.vi"("Reply (F)"=TRUE, "error in (no error)"=w16) -> ("error out"=w2:errorcluster)  [unwired: 9 in]
  "error out" <- w2
  n190 = case "External Launch?" shown="True" w5 {
    tunnel: w2 -> [_ w382]
    frame False {
    }
    frame True {
      n191 = case shown="No Error" w382 {
        frame No Error {
          n192 = invoke on="Invoke Node" class="VI" method="FP.Close"() -> ()  [unwired: 3 in, 3 out]
        }
        frame Error {
          n193 = invoke on="Invoke Node" class="VI" method="FP.Open"("Activate"=TRUE ("Activate?")) -> ()  [unwired: 4 in, 5 out]
        }
      }
    }
  }
  n194 = local write "Module Admin"(w6) -> ()
